vi "Plot_to_file.vi"(6 "Show Smooth":bool, 7 "Start trace No":i32, 8 "Trace names":string[](array[string]), 9 "Graph":T2={"Plot 1"=1, "Plot 2"=3, "Save graph"=0, "Plot Type"=enum."Voltage trace"} {"Save graph" items=["Do not save plot", "Save plot"]; "Plot 2" items=["Nothing", "Velocity1", "Arr time1", "Velocity2", "Arr time2"]; "Plot 1" items=["Nothing", "Velocity1", "Arr time1", "Velocity2", "Arr time2"]}, 10 "Plot file label":string[][](array[string]), 11 "Plot data":cluster{"Xo":dbl, "Delta X":dbl, dbl[]}[](array[cluster]) {"?" format="%.2f"; "Delta X" format="%.2f"; "Xo" format="%.2f"}) -> (3 "End trace No":i32)   [LabVIEW 2020]
uses:
  Globals/Meas_global.vi
  Controls/Graph_Type.ctl
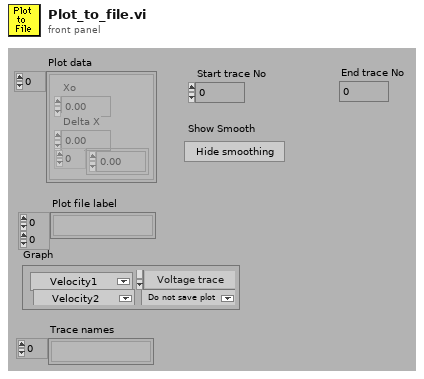
[diagram p1: front panel]
types:
  T1 = typedef "Graph_Type.ctl" = enum16{"Show no graph", "Voltage trace", "Velocity trace", "Vel histogram", "Spectrum", "f.E(f) v Log f", "Auto-Corr"}
  T2 = cluster{"Plot 1":u16, "Plot 2":u16, "Save graph":u16, "Plot Type":T1}
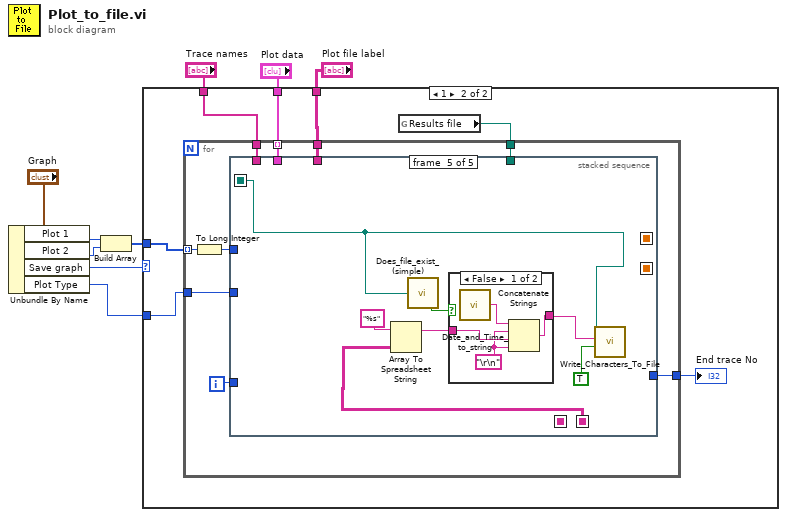
[diagram p0: block diagram]
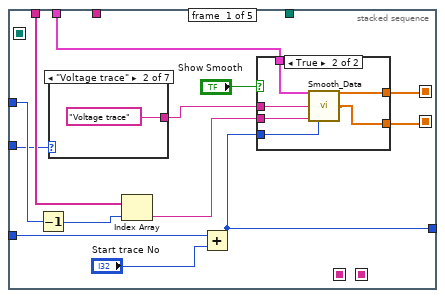
[diagram p3: hidden frame]
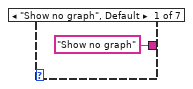
[diagram p4: hidden frame]
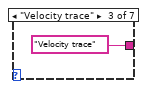
[diagram p5: hidden frame]
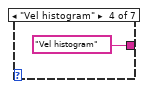
[diagram p6: hidden frame]
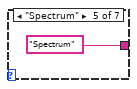
[diagram p7: hidden frame]
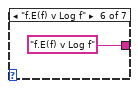
[diagram p8: hidden frame]
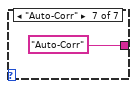
[diagram p9: hidden frame]
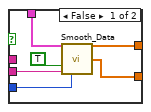
[diagram p10: hidden frame]
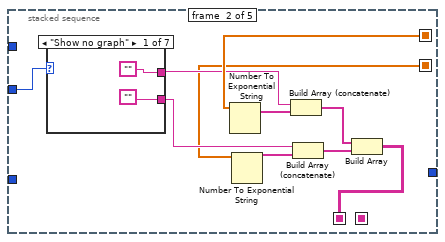
[diagram p11: hidden frame]
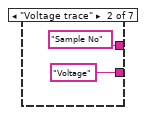
[diagram p12: hidden frame]
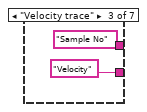
[diagram p13: hidden frame]
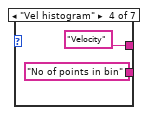
[diagram p14: hidden frame]
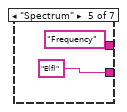
[diagram p15: hidden frame]
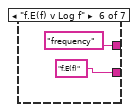
[diagram p16: hidden frame]
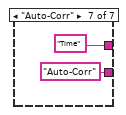
[diagram p17: hidden frame]
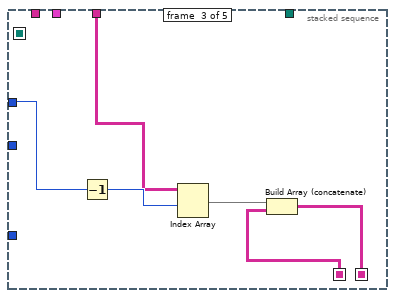
[diagram p18: hidden frame]
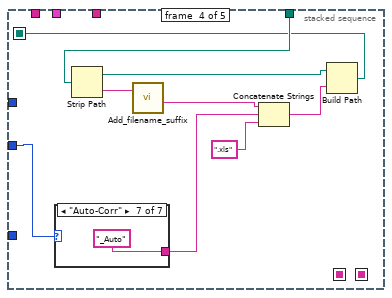
[diagram p19: hidden frame]
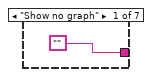
[diagram p20: hidden frame]
diagram:
  n1 = Unbundle By Name("Graph") -> ("Plot 1"=w4:u16, "Plot 2"=w3:u16, "Save graph"=w7:u16, "Plot Type"=w6:T1)
  n2 = Build Array(w4, w3) -> (w2:u16[])
  n3 = case shown="1" w7 {
    tunnel: "Plot data" -> [_ w16]
    tunnel: w6 -> [_ w15]
    tunnel: "Plot file label" -> [_ w14]
    tunnel: w2 -> [_ w13]
    tunnel: "Trace names" -> [_ w10]
    frame 0, Default {
    }
    frame 1 {
      n4 = global read "Meas_global.vi" "Results file"() -> (w11:path)
      n5 = for {
        tunnel: w15 -> [w22]
        tunnel: w13 -> [w25] mode=indexing
        tunnel: w14 -> [w24]
        tunnel: w16 -> [w23] mode=indexing
        tunnel: [w20] -> w12
        tunnel: w11 -> [w19]
        tunnel: w10 -> [w18]
        i -> [w21]
        n6 = To Long Integer(number=w25) -> (32bit integer=w17:i32)
        n7 = stacked-sequence {
          seq-local: [_ _ w82 _ _] -> [_ _ _ _ w105]
          seq-local: [w30 _ _ _ _] -> [_ w62 _ _ _]
          seq-local: [w29 _ _ _ _] -> [_ w59 _ _ _]
          seq-local: [_ w58 _ _ _] -> [_ _ w83 _ _]
          seq-local: [_ _ _ w88 _] -> [_ _ _ _ w104]
          tunnel: w17 -> [w38 _ w85 _ _]
          tunnel: w24 -> [_ _ w86 _ _]
          tunnel: w23 -> [w37 _ _ _ _]
          tunnel: w22 -> [w28 w63 _ w95 _]
          tunnel: w21 -> [w35 _ _ _ _]
          tunnel: [w34 _ _ _ _] -> w20
          tunnel: w19 -> [_ _ _ w96 _]
          tunnel: w18 -> [w32 _ _ _ _]
          frame #0 {
            n8 = Decrement(x=w38) -> (x-1=w33:i32)
            n9 = case shown="\"Voltage trace\"" w28 {
              tunnel: ["Show no graph" "Voltage trace" "Velocity trace" "Vel histogram" "Spectrum" "f.E(f) v Log f" "Auto-Corr"] -> w27
              frame "Show no graph", Default {
              }
              frame "Voltage trace" {
              }
              frame "Velocity trace" {
              }
              frame "Vel histogram" {
              }
              frame "Spectrum" {
              }
              frame "f.E(f) v Log f" {
              }
              frame "Auto-Corr" {
              }
            }
            n10 = Index Array(array=w32, index=w33) -> (element=w31:string)
            n11 = Add(x=w35, y="Start trace No") -> (x+y=w34:i32)
            n12 = case shown="True" "Show Smooth" {
              tunnel: w37 -> [w51 w57]
              tunnel: w34 -> [w49 w56]
              tunnel: w31 -> [w48 w55]
              tunnel: [w47 w54] -> w30
              tunnel: [w46 w53] -> w29
              tunnel: w27 -> [_ w52]
              frame False {
                n13 = call "Smooth_Data.vi"("Plot cluster"=w51, "OK"=TRUE, "Trace name"=w48, "Trace No"=w49) -> ("X array Out"=w47:dbl[], "Y array Out"=w46:dbl[])  [unwired: 2 in, 8 out]
              }
              frame True {
                n14 = call "Smooth_Data.vi"("Plot cluster"=w57, "Plot type"=w52, "Trace name"=w55, "Trace No"=w56) -> ("X array Out"=w54:dbl[], "Y array Out"=w53:dbl[])  [unwired: 2 in, 8 out]
              }
            }
          }
          frame #1 {
            n15 = case shown="\"Show no graph\"" w63 {
              tunnel: ["" "Sample No" "Sample No" "Velocity" "Frequency" "frequency" "Time"] -> w61
              tunnel: ["" "Voltage" "Velocity" "No of points in bin" "E(f)" "f.E(f)" "Auto-Corr"] -> w60
              frame "Show no graph" {
              }
              frame "Voltage trace" {
              }
              frame "Velocity trace" {
              }
              frame "Vel histogram" {
              }
              frame "Spectrum" {
              }
              frame "f.E(f) v Log f" {
              }
              frame "Auto-Corr" {
              }
            }
            n16 = Number To Exponential String(number=w62) -> (E-format string=w66:string[])  [unwired: 3 out]
            n17 = Number To Exponential String(number=w59) -> (E-format string=w67:string[])  [unwired: 3 out]
            n18 = Build Array (concatenate)(w61, w66) -> (w64:string[])
            n19 = Build Array (concatenate)(w60, w67) -> (w65:string[])
            n20 = Build Array(w64, w65) -> (w58:string[][])
          }
          frame #2 {
            n21 = Decrement(x=w85) -> (x-1=w87:i32)
            n22 = Index Array(array=w86, index (row)=w87) -> (element=w84:string[])  [unwired: 1 in]
            n23 = Build Array (concatenate)(w84, w83) -> (w82:string[][])
          }
          frame #3 {
            n24 = case shown="\"Auto-Corr\"" w95 {
              tunnel: ["" "_Volt" "_Vel" "_Hist" "_Spec" "_f.E(f)" "_Auto"] -> w92
              frame "Show no graph" {
              }
              frame "Voltage trace" {
              }
              frame "Velocity trace" {
              }
              frame "Vel histogram" {
              }
              frame "Spectrum" {
              }
              frame "f.E(f) v Log f" {
              }
              frame "Auto-Corr" {
              }
            }
            n25 = Strip Path(path=w96) -> (stripped path=w89:path, name=w94:string)
            n26 = call "Add_filename_suffix.vi"("Filename"=w94) -> ("Base name"=w93:string)  [unwired: 1 in, 3 out]
            n27 = Concatenate Strings(w93, w92, ".xls" ("string")) -> (w90:string)
            n28 = Build Path(base path=w89, name or relative path=w90) -> (appended path=w88:path)
          }
          frame #4 {
            n29 = Array To Spreadsheet String(array=w105, 3:"%s") -> (spreadsheet string=w107:string)  [unwired: 1 out]
            n30 = call "Does_file_exist_(simple).vi"("Pathname"=w104) -> ("exists?"=w106:bool)
            n31 = case shown="False" w106 {
              tunnel: w107 -> [w114 w117]
              tunnel: [w112 w116] -> w108
              frame False {
                w113 = "\r\n"
                n32 = call "Date_and_Time_to_string.vi"() -> ("Date and time (spreadsheet)"=w111:string)  [unwired: 4 in, 1 out]
                n33 = Concatenate Strings(w111, w113, w114, w113) -> (w112:string)
              }
              frame True {
                n34 = Concatenate Strings(w117, "\r\n") -> (w116:string)
              }
            }
            n35 = call "Write_Characters_To_File.vi"("file path (dialog if empty)"=w104, "character string"=w108, "append to file? (new file:F)"=TRUE) -> ()  [unwired: 2 in, 4 out]
          }
        }
      }
      "End trace No" <- w12
    }
  }
